vi "Write All.vi"(8 "Error In":errorcluster, 10 "Data":u8[](array[numeric]), 11 "Channel In":refnum<class "Channel.lvclass">=refnum) -> (0 "Error Out":errorcluster, 1 "Timed Out?":bool, 2 "Write Count":u64, 3 "Channel Out":refnum<class "Channel.lvclass">)   [LabVIEW 2021, in "Field_RnD_Services_LIBSSH2_Toolkit.lvlib" / "Channel.lvclass"]
doc: "Writes binary data to the SSH channel represented by this Channel object until all of the data (bytes) are written. If the binary data is larger than 30KB, then the data is written in 30KB chunks, or blocks, until the <B>Write Count</B> equals the <B>Data</B> array size."
uses:
  Channel.lvclass
  Channel.lvclass/Channel.ctl
  Session/Session.lvclass
  SSH/SSH.lvclass
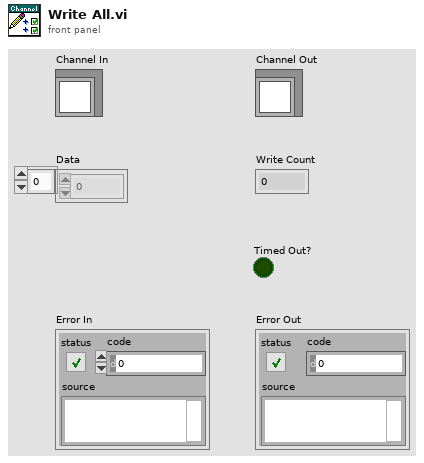
[diagram p1: front panel]
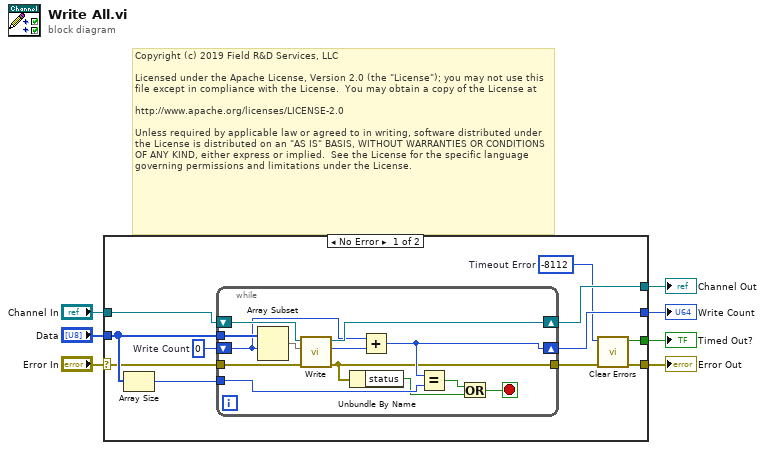
[diagram p0: block diagram]
diagram:
  # "Copyright (c) 2019 Field R&D Services, LLC\n\nLicensed under the Apache License, Version 2.0 (the \"License\"); you may not use this file except in compliance with the License.  You may obtain a copy of the License at\n\nhttp://www.apache.org/licenses/LICENSE-2.0\n\nUnless required by applicable law or agreed to in writing, software distributed under the License is distributed on an \"AS IS\" BASIS, WITHOUT WARRANTIES OR CONDITIONS OF ANY KIND, either express or implied.  See the License for the specific language governing permissions and limitations under the License."
  n1 = case shown="No Error" "Error In" {
    selector: "Error In" -> [w12 w32]
    tunnel: "Data" -> [w16 _]
    tunnel: "Channel In" -> [w15 w33]
    tunnel: [w14 w33] -> w5
    tunnel: [w10 w32] -> w4
    tunnel: [w11 _] -> w2
    tunnel: [w8 _] -> w1
    frame No Error {
      w9 = -8112  # Timeout Error
      w17 = u64 0  # Write Count
      n2 = Array Size(array=w16) -> (size(s)=w18:i32)
      n3 = while {
        tunnel: w16 -> [w28]
        shift-right: [w29] -> w14
        shift-left: w15 -> [w30]
        tunnel: w18 -> [w23]
        shift-right: [w24] -> w11
        shift-left: w17 -> [w25]
        tunnel: w12 -> [w31]
        tunnel: [w21] -> w13
        stop <- w19 stop-if-true
        n4 = Array Subset(array=w28, index=w25) -> (w27:u8[])  [unwired: 1 in]
        n5 = call "Write.vi"("Error In"=w31, "Data"=w27, "Channel In"=w30) -> ("Error Out"=w21:errorcluster, "Write Count"=w26:u64, "Channel Out"=w29:refnum<class "Channel.lvclass">)  [unwired: 6 in]
        n6 = Unbundle By Name(w21) -> ("status"=w20:bool)
        n7 = Add(x=w25, y=w26) -> (x+y=w24:u64)
        n8 = Equal?(x=w24, y=w23) -> (x = y?=w22:bool)
        n9 = Or(x=w22, y=w20) -> (x .or. y?=w19:bool)
      }
      n10 = call <vilib>:"Clear Errors.vi"("error in (no error)"=w13, "specific error code to clear (0: all)"=w9) -> ("error out"=w10:errorcluster, "specific error cleared?"=w8:bool)  [unwired: 4 in]
    }
    frame Error {
    }
  }
  "Channel Out" <- w5
  "Error Out" <- w4
  "Write Count" <- w2
  "Timed Out?" <- w1
